vi "读取返回数据事件.vi"(8 "error in (no error)":errorcluster caption="错误输入（无错误）", 11 "通讯输入":refnum<class "通讯.lvclass">) -> (0 "error out":errorcluster caption="错误输出", 2 "返回数据事件":refnum<user-event>, 3 "通讯输出":refnum<class "通讯.lvclass">)   [LabVIEW 2015, in "通讯.lvlib" / "通讯.lvclass"]
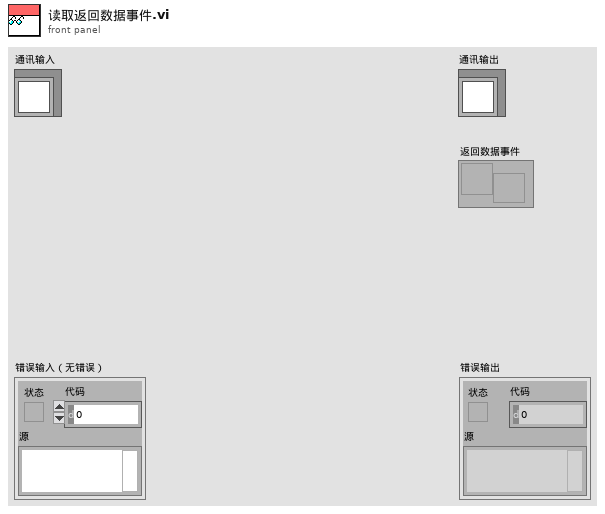
[diagram p1: front panel]
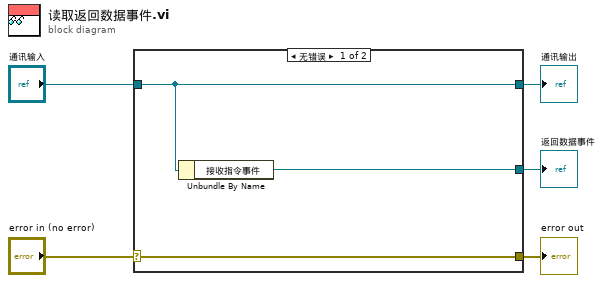
[diagram p0: block diagram]
diagram:
  n1 = case shown="无错误" "error in (no error)" {
    selector: "error in (no error)" -> [w8 w9]
    tunnel: [w8 w9] -> w4
    tunnel: [w7 w10] -> w2
    tunnel: "通讯输入" -> [w7 w10]
    tunnel: [w6 _] -> w1
    frame No Error {
      n2 = Unbundle By Name(w7) -> ("接收指令事件"=w6:refnum<user-event>)
    }
    frame Error {
    }
  }
  "error out" <- w4
  "通讯输出" <- w2
  "返回数据事件" <- w1
